vi "queue.vi"() -> ()   [LabVIEW 2017]
panel:
  in  "milliseconds to wait 2":u32
  out "Waveform Chart 2":dbl(graph)
  in  "Stop Button 2":bool
  in  "milliseconds to wait":u32
  out "Waveform Chart":dbl(graph)
  in  "Stop Button":bool
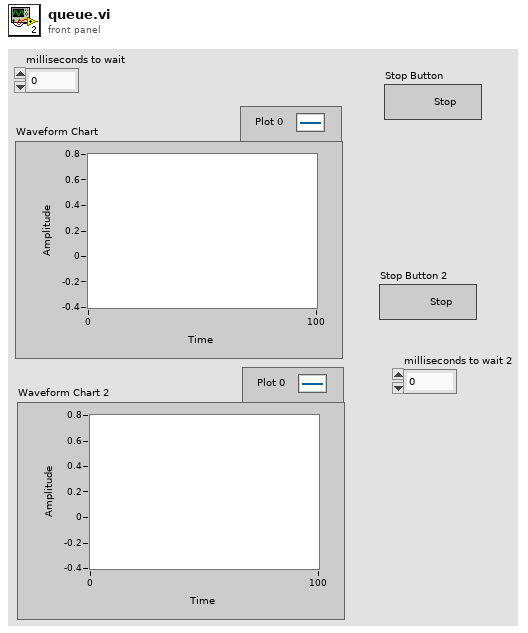
[diagram p1: front panel]
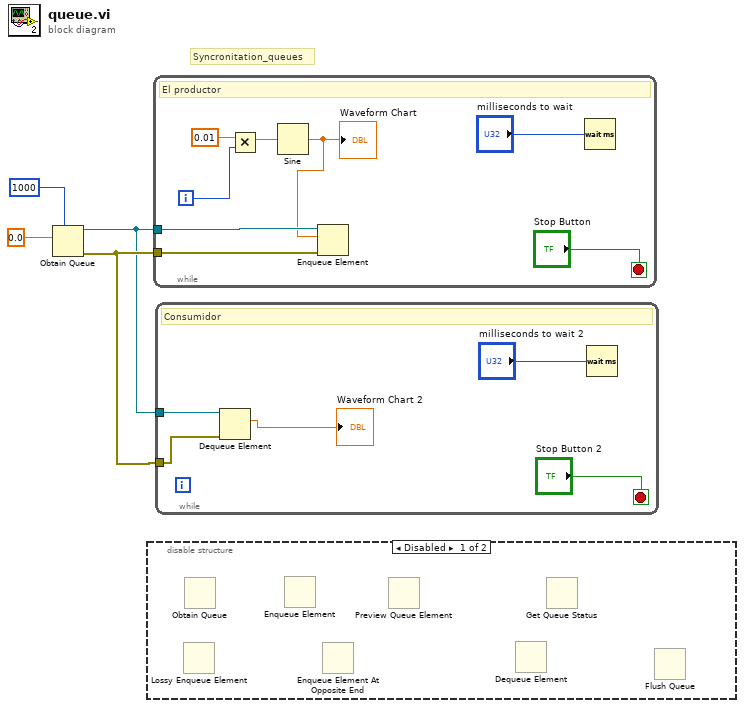
[diagram p0: block diagram]
diagram:
  # "Syncronitation_queues"
  n1 = Obtain Queue(max queue size (-1, unlimited)=1000, element data type=0.0) -> (queue out=w1:refnum<queue>, error out=w2:errorcluster)  [unwired: 3 in, 1 out]
  n2 = disable-structure shown="Disabled" {
    frame Disabled {
      n3 = Lossy Enqueue Element() -> ()  [unwired: 3 in, 4 out]
      n4 = Obtain Queue() -> ()  [unwired: 5 in, 3 out]
      n5 = Enqueue Element() -> ()  [unwired: 4 in, 3 out]
      n6 = Enqueue Element At Opposite End() -> ()  [unwired: 4 in, 3 out]
      n7 = Preview Queue Element() -> ()  [unwired: 3 in, 4 out]
      n8 = Dequeue Element() -> ()  [unwired: 3 in, 4 out]
      n9 = Get Queue Status() -> ()  [unwired: 3 in, 8 out]
      n10 = Flush Queue() -> ()  [unwired: 2 in, 3 out]
    }
    frame Enabled {
    }
  }
  n11 = while {
    tunnel: w2 -> [w7]
    tunnel: w1 -> [w6]
    i -> [w10]
    stop <- "Stop Button" stop-if-true
    # "El productor"
    n12 = Multiply(x=0.01, y=w10) -> (x*y=w9:dbl)
    n13 = Sine(x=w9) -> (sin(x)=w5:dbl)
    "Waveform Chart" <- w5
    n14 = Enqueue Element(queue=w6, element=w5, error in (no error)=w7) -> ()  [unwired: 1 in, 3 out]
    n15 = Wait (ms)(milliseconds to wait="milliseconds to wait") -> ()  [unwired: 1 out]
  }
  n16 = while {
    tunnel: w2 -> [w15]
    tunnel: w1 -> [w14]
    stop <- "Stop Button 2" stop-if-true
    # "Consumidor"
    n17 = Dequeue Element(queue=w14, error in (no error)=w15) -> (element=→"Waveform Chart 2":dbl)  [unwired: 1 in, 3 out]
    n18 = Wait (ms)(milliseconds to wait="milliseconds to wait 2") -> ()  [unwired: 1 out]
  }
